vi "BASE_Create Login.vi"(6 "Error In":errorcluster, 8 "Password":string, 9 "User Name":string(combo)) -> (0 "error out":errorcluster)   [LabVIEW 2017]
uses:
  <vilib>/Utility/config.llb/Write Key (String).vi
  <vilib>/Utility/config.llb/Write Key (I32).vi
  <vilib>/Utility/config.llb/NI_LVConfig.lvlib
panel:
  in  "Level":u16(ring) items=["", "Operator", "Superviser", "Admin"]
  in  "Delete":bool
  in  "Exit":bool
  in  "Create":bool
  # "CREATE LOGIN"
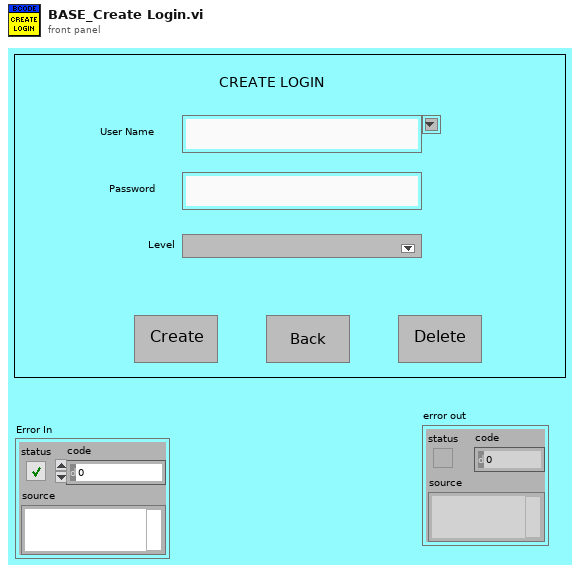
[diagram p1: front panel]
types:
  T1 = enum32{"invalid app kind", "Development System", "Run Time System", "Student Edition", "Embedded LabVIEW", "Evaluation", "Custom"}
  T2 = typedef "NI_LVConfig.lvlib/Config Data RefNum.ctl" = refnum<k1>
  T3 = enum32{"Invalid", "Standard", "Closed", "Hidden", "Minimized", "Maximized"}
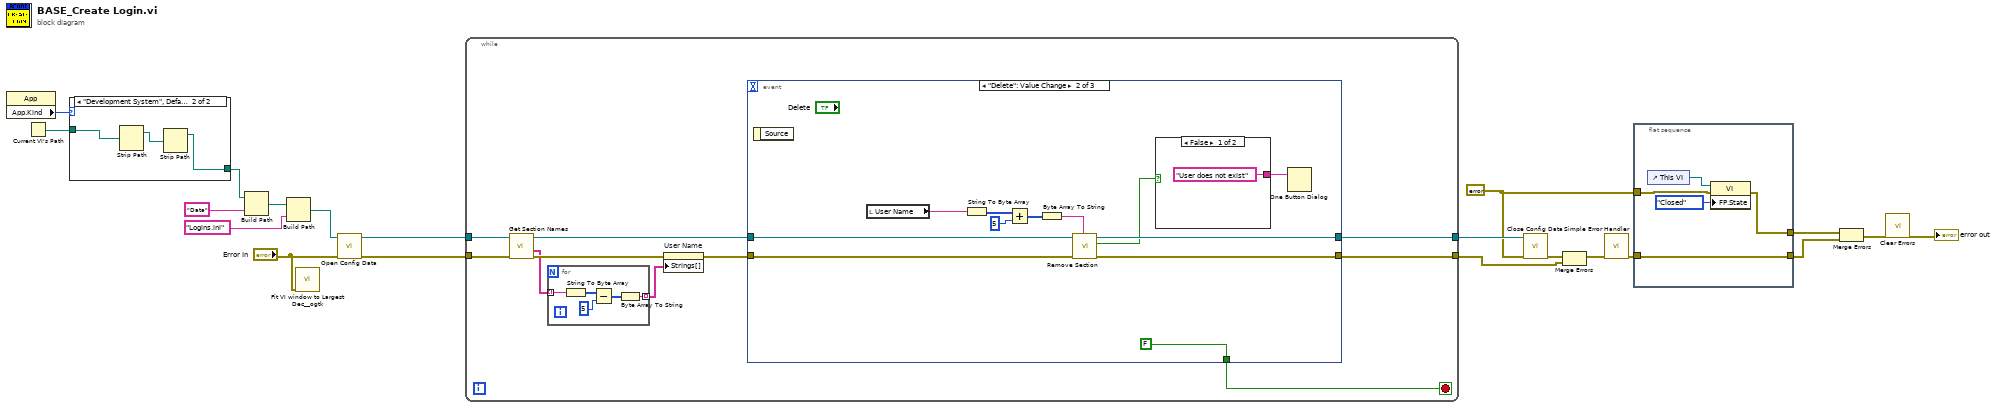
[diagram p0: block diagram]
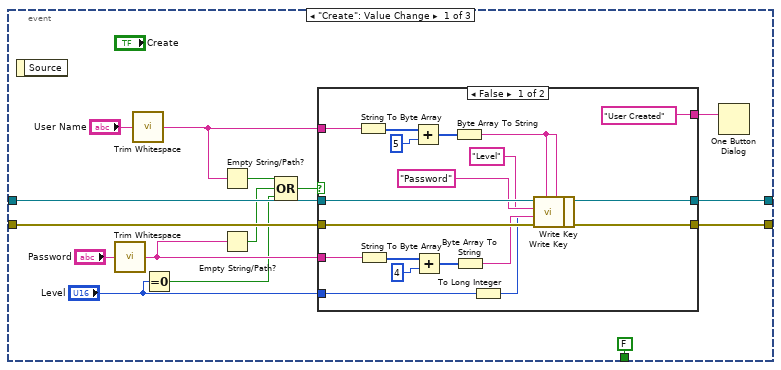
[diagram p2: hidden frame]
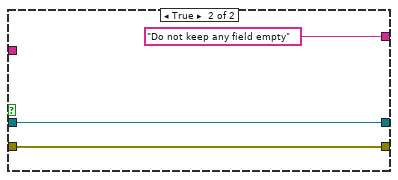
[diagram p3: hidden frame]
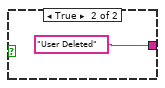
[diagram p4: hidden frame]
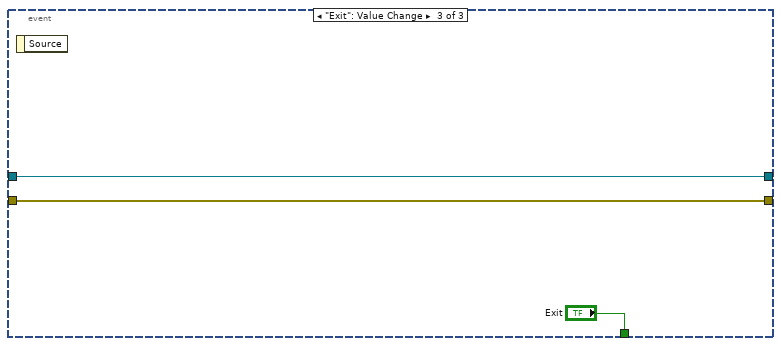
[diagram p5: hidden frame]
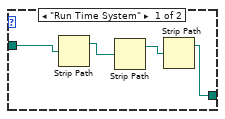
[diagram p6: hidden frame]
diagram:
  w11 = errorcluster {"status"=FALSE, "code"=0, "source"=""} ("error in (no error)")
  n1 = property class="App"() -> ("App.Kind"=w19:T1)  [unwired: 2 in, 2 out]
  n2 = Current VI's Path() -> (path=w20:path)
  n3 = case shown="\"Development System\", Default" w19 {
    tunnel: w20 -> [w22 w26]
    tunnel: [w21 w25] -> w17
    frame "Run Time System" {
      n4 = Strip Path(path=w22) -> (stripped path=w24:path)  [unwired: 1 out]
      n5 = Strip Path(path=w24) -> (stripped path=w23:path)  [unwired: 1 out]
      n6 = Strip Path(path=w23) -> (stripped path=w21:path)  [unwired: 1 out]
    }
    frame "Development System", Default {
      n7 = Strip Path(path=w26) -> (stripped path=w27:path)  [unwired: 1 out]
      n8 = Strip Path(path=w27) -> (stripped path=w25:path)  [unwired: 1 out]
    }
  }
  n9 = Build Path(base path=w17, name or relative path="Data") -> (appended path=w18:path)
  n10 = Build Path(base path=w18, name or relative path="Logins.ini") -> (appended path=w16:path)
  n11 = call <userlib>:"Fit VI window to Largest Dec__ogtk.vi"("error in (no error)"="Error In") -> ()  [unwired: 5 in, 2 out]
  n12 = call <vilib>:"Open Config Data.vi"("error in (no error)"="Error In", "configuration file path"=w16) -> ("error out"=w5:errorcluster, "refnum"=w4:T2)  [unwired: 7 in, 1 out]
  n13 = while {
    tunnel: [w37] -> w2
    tunnel: [w36] -> w13
    tunnel: w5 -> [w34]
    tunnel: w4 -> [w33]
    stop <- w35 stop-if-true
    n14 = call <vilib>:"Get Section Names.vi"("error in (no error)"=w34, "refnum"=w33) -> ("error out"=w31:errorcluster, "section names"=w29:string[], "refnum out"=w32:T2)  [unwired: 7 in]
    n15 = for {
      tunnel: w29 -> [w98] mode=indexing
      tunnel: [w94] -> w28 mode=indexing
      n16 = String To Byte Array(string=w98) -> (unsigned byte array=w97:u8[])
      n17 = Subtract(x=w97, y=u8 5) -> (x-y=w95:u8[])
      n18 = Byte Array To String(unsigned byte array=w95) -> (string=w94:string)
    }
    n19 = property on="User Name" class="CmbBox"(error in=w31, "Strings[]"=w28) -> (error out=w30:errorcluster)  [unwired: 1 in, 1 out]
    n20 = event shown="[1] \"Delete\": Value Change" {
      selector: _ -> [_ _ _]
      dyn-events: _ -> [_ _ _]
      timeout: _ -> [_ _ _]
      tunnel: w32 -> [w52 w88 w92]
      tunnel: w30 -> [w51 w87 w91]
      tunnel: [w48 w85 w91] -> w37
      tunnel: [w49 w86 w92] -> w36
      tunnel: [FALSE ("Exit") FALSE ("Exit") "Exit"] -> w35
      event "Create": Value Change {
        n21 = event-data() -> ()  [unwired: 1 in, 1 out]
        n22 = call <vilib>:"Trim Whitespace.vi"("string"="Password") -> ("trimmed string"=w41:string)  [unwired: 1 in]
        n23 = call <vilib>:"Trim Whitespace.vi"("string"="User Name") -> ("trimmed string"=w42:string)  [unwired: 1 in]
        n24 = Equal To 0?(x="Level") -> (x = 0?=w39:bool)
        n25 = Empty String/Path?(string/path=w42) -> (empty?=w47:bool)
        n26 = Empty String/Path?(string/path=w41) -> (empty?=w46:bool)
        n27 = Compound Arithmetic op=OR(w47, w46, w39) -> (w45:bool)
        n28 = case shown="False" w45 {
          tunnel: w52 -> [w73 w76]
          tunnel: w51 -> [w72 w75]
          tunnel: [w58 w76] -> w49
          tunnel: [w60 w75] -> w48
          tunnel: w42 -> [w62 _]
          tunnel: w41 -> [w70 _]
          tunnel: "Level" -> [w54 _]
          tunnel: ["User Created" ("message") "Do not keep any field empty" ("message")] -> w38
          frame False {
            n29 = String To Byte Array(string=w62) -> (unsigned byte array=w63:u8[])
            n30 = String To Byte Array(string=w70) -> (unsigned byte array=w69:u8[])
            n31 = Add(x=w63, y=u8 5) -> (x+y=w65:u8[])
            n32 = Add(x=w69, y=u8 4) -> (x+y=w67:u8[])
            n33 = Byte Array To String(unsigned byte array=w65) -> (string=w57:string)
            n34 = Byte Array To String(unsigned byte array=w67) -> (string=w66:string)
            n35 = To Long Integer(number=w54) -> (32bit integer=w55:i32)
            n36 = call-poly <vilib>:"Write Key.vi"("section"=w57, "error in (no error)"=w72, "value"=w66, "key"="Password", "refnum"=w73) -> ("error out"=w61:errorcluster, "refnum out"=w59:T2)  [unwired: 4 in, 1 out]
            n37 = call-poly <vilib>:"Write Key.vi"("section"=w57, "error in (no error)"=w61, "value"=w55, "key"="Level", "refnum"=w59) -> ("error out"=w60:errorcluster, "refnum out"=w58:T2)  [unwired: 4 in, 1 out]
          }
          frame True {
          }
        }
        n38 = One Button Dialog(message=w38) -> ()  [unwired: 1 in, 1 out]
      }
      event "Delete": Value Change {
        n39 = event-data() -> ()  [unwired: 1 in, 1 out]
        n40 = local read "User Name"() -> (w80:string)
        n41 = String To Byte Array(string=w80) -> (unsigned byte array=w81:u8[])
        n42 = Add(x=w81, y=u8 5) -> (x+y=w83:u8[])
        n43 = Byte Array To String(unsigned byte array=w83) -> (string=w79:string)
        n44 = call <vilib>:"Remove Section.vi"("section"=w79, "error in (no error)"=w87, "refnum"=w88) -> ("error out"=w85:errorcluster, "section exists?"=w78:bool, "refnum out"=w86:T2)  [unwired: 6 in]
        n45 = case shown="False" w78 {
          tunnel: ["User does not exist" ("message") "User Deleted" ("message")] -> w77
          frame False {
          }
          frame True {
          }
        }
        n46 = One Button Dialog(message=w77) -> ()  [unwired: 1 in, 1 out]
      }
      event "Exit": Value Change {
        n47 = event-data() -> ()  [unwired: 1 in, 1 out]
      }
    }
  }
  n48 = call <vilib>:"Close Config Data.vi"("error in (no error)"=w11, "refnum"=w13) -> ("error out"=w12:errorcluster)  [unwired: 8 in, 1 out]
  n49 = Merge Errors(w12, w2) -> (w3:errorcluster)
  n50 = call <vilib>:"Simple Error Handler.vi"("error in (no error)"=w3) -> ("error out"=w6:errorcluster)  [unwired: 4 in, 4 out]
  n51 = flat-sequence {
    tunnel: w11 -> [w101]
    tunnel: [w100] -> w10
    tunnel: [w99] -> w7
    tunnel: w6 -> [w99]
    frame #0 {
      n52 = control-ref of="This VI"() -> (w103:refnum<vi>)
      n53 = property class="VI"(reference=w103, error in=w101, "FP.State"=T3."Closed" ("Front Panel Window:State")) -> (error out=w100:errorcluster)  [unwired: 1 out]
    }
  }
  n54 = Merge Errors(w10, w7) -> (w9:errorcluster)
  n55 = call <vilib>:"Clear Errors.vi"("error in (no error)"=w9) -> ("error out"=→"error out":errorcluster)  [unwired: 5 in, 1 out]
